vi "校准_数据库操作.vi"(8 "error in (no error)":errorcluster, 9 "出口":i32, 10 "进口":i32, 11 "Freq&S":T1) -> (0 "error out":errorcluster)   [LabVIEW 2015]
uses:
  network_Global/Global.vi
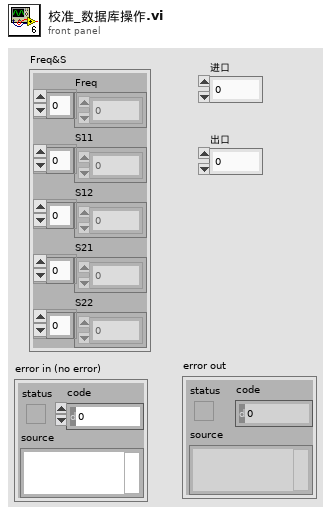
[diagram p1: front panel]
types:
  T1 = cluster{"Freq":dbl[], "S11":dbl[], "S12":dbl[], "S21":dbl[], "S22":dbl[]}
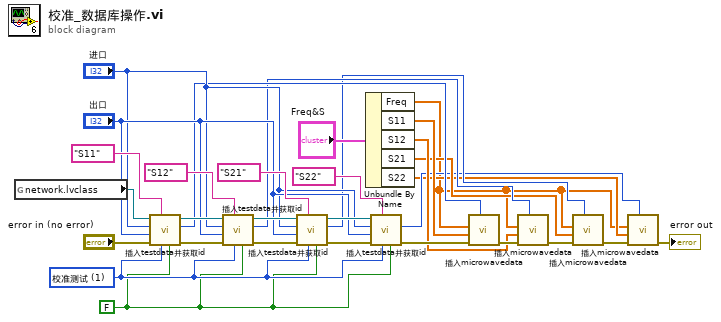
[diagram p0: block diagram]
diagram:
  w3 = FALSE ("Ref")
  w4 = u16 1 items=["直通测试", "校准测试", "电缆"] ("测试类型")
  n1 = global read "Global.vi" "network.lvclass"() -> (w31:refnum<class "network.lvclass">)
  n2 = call "插入testdata并获取id.vi"("Ref"=w3, "测试类型"=w4, "数据类型"="S11" ("Combo Box"), "error in (no error)"="error in (no error)", "出口"="出口", "进口"="进口", "network in"=w31) -> ("error out"=w22:errorcluster, "id"=w17:i32, "network out"=w23:refnum<class "network.lvclass">)  [unwired: 2 in]
  n3 = call "插入testdata并获取id.vi"("Ref"=w3, "测试类型"=w4, "数据类型"="S12" ("Combo Box"), "error in (no error)"=w22, "出口"="出口", "进口"="进口", "network in"=w23) -> ("error out"=w25:errorcluster, "id"=w12:i32, "network out"=w24:refnum<class "network.lvclass">)  [unwired: 2 in]
  n4 = call "插入testdata并获取id.vi"("Ref"=w3, "测试类型"=w4, "数据类型"="S21" ("Combo Box"), "error in (no error)"=w25, "出口"="出口", "进口"="进口", "network in"=w24) -> ("error out"=w27:errorcluster, "id"=w9:i32, "network out"=w26:refnum<class "network.lvclass">)  [unwired: 2 in]
  n5 = Unbundle By Name("Freq&S") -> ("Freq"=w5:dbl[], "S11"=w14:dbl[], "S12"=w13:dbl[], "S21"=w10:dbl[], "S22"=w6:dbl[])
  n6 = call "插入testdata并获取id.vi"("Ref"=w3, "测试类型"=w4, "数据类型"="S22" ("Combo Box"), "error in (no error)"=w27, "出口"="出口", "进口"="进口", "network in"=w26) -> ("error out"=w18:errorcluster, "id"=w8:i32)  [unwired: 2 in, 1 out]
  n7 = call "插入microwavedata.vi"("pid"=w17, "error in"=w18, "S-Parameter"=w14, "freq"=w5) -> ("error out"=w15:errorcluster)  [unwired: 7 in]
  n8 = call "插入microwavedata.vi"("pid"=w12, "error in"=w15, "S-Parameter"=w13, "freq"=w5) -> ("error out"=w11:errorcluster)  [unwired: 7 in]
  n9 = call "插入microwavedata.vi"("pid"=w9, "error in"=w11, "S-Parameter"=w10, "freq"=w5) -> ("error out"=w7:errorcluster)  [unwired: 7 in]
  n10 = call "插入microwavedata.vi"("pid"=w8, "error in"=w7, "S-Parameter"=w6, "freq"=w5) -> ("error out"=→"error out":errorcluster)  [unwired: 7 in]
